vi "LVClass_CorrectionDataManager GetWavefrontCorrectorInitialPreferences.vi"(0 "CorrectionDataManager in":refnum<class "CorrectionDataManager.lvclass">, 11 "error in (no error)":errorcluster) -> (4 "CorrectionDataManager out":refnum<class "CorrectionDataManager.lvclass">, 8 "Wavefront Corrector State":T1[](array[typedef]), 15 "error out":errorcluster)   [LabVIEW 2020, in "CorrectionDataManager.lvclass"]
doc: "--------------------------------------------------------------------------------\n\n<B>corrdata_managerIn </B> : CorrDataManager object\n<B>corrdata_managerOut </B> : CorrDataManager object\n<B>min </B> : WavefrontCorrector preferences : lowest command value.\n<B>max </B> : WavefrontCorrector preferences : highest command value.\n<B>validity </B> : WavefrontCorrector preferences : status.\n<B>fixed_value </B> : WavefrontCorrector preferences : fixed positions.\n<B>ErrorIn </B> : Error\n<B>ErrorOut </B> : Error\n\n--------------------------------------------------------------------------------"
uses:
  CorrectionDataManager.lvclass
  Wavefront Corrector states - ONE.ctl
  CorrectionDataManager.lvclass/CorrectionDataManager.ctl
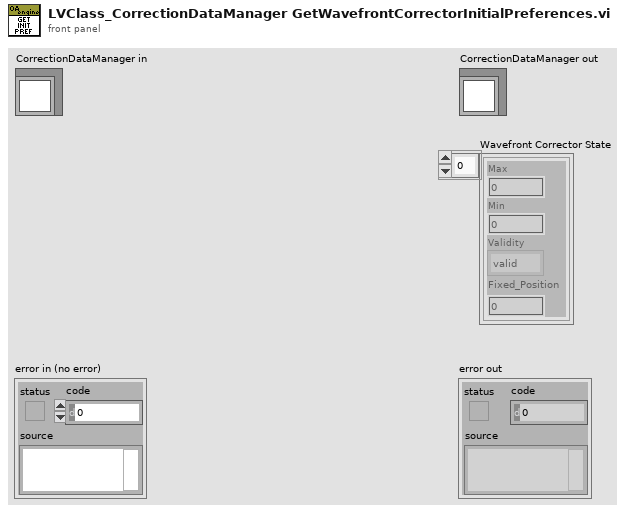
[diagram p1: front panel]
types:
  T1 = typedef "Wavefront Corrector states - ONE.ctl" = cluster{"Max":sgl, "Min":sgl, "Validity":enum16{"valid", "fixed", "invalid"}, "Fixed_Position":sgl}
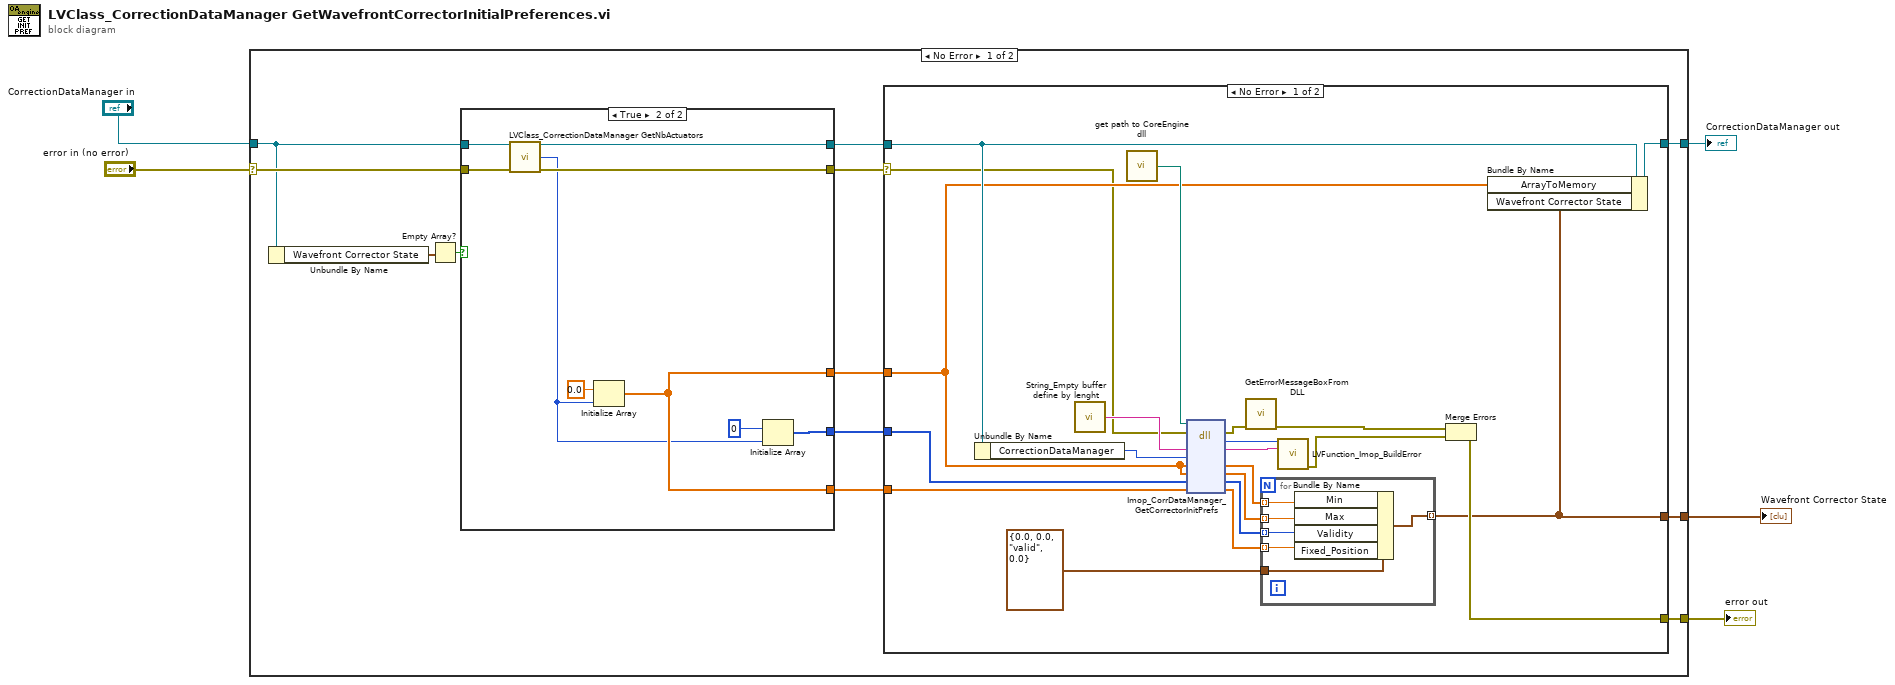
[diagram p0: block diagram]
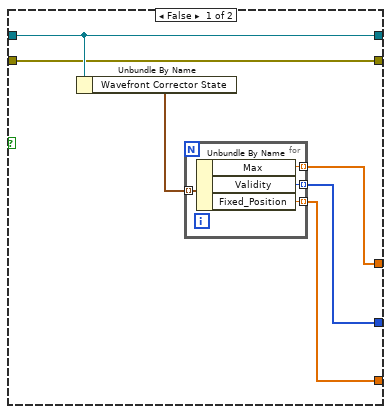
[diagram p3: hidden frame]
diagram:
  n1 = case shown="No Error" "error in (no error)" {
    selector: "error in (no error)" -> [w14 w67]
    tunnel: [w17 w67] -> w4
    tunnel: [w9 w66] -> w5
    tunnel: "CorrectionDataManager in" -> [w13 w66]
    tunnel: [w8 _] -> w1
    frame No Error {
      n2 = Unbundle By Name(w13) -> ("Wavefront Corrector State"=w16:T1[])
      n3 = Empty Array?(array=w16) -> (empty?=w15:bool)
      n4 = case shown="True" w15 {
        tunnel: w13 -> [w52 w63]
        tunnel: [w52 w57] -> w10
        tunnel: [w50 w59] -> w7
        tunnel: [w48 w59] -> w12
        tunnel: w14 -> [w51 w62]
        tunnel: [w51 w61] -> w6
        tunnel: [w49 w60] -> w11
        frame False {
          n5 = Unbundle By Name(w52) -> ("Wavefront Corrector State"=w47:T1[])
          n6 = for {
            tunnel: w47 -> [w56] mode=indexing
            tunnel: [w55] -> w50 mode=indexing
            tunnel: [w54] -> w49 mode=indexing
            tunnel: [w53] -> w48 mode=indexing
            n7 = Unbundle By Name(w56) -> ("Max"=w55:sgl, "Validity"=w54:enum16{"valid", "fixed", "invalid"}, "Fixed_Position"=w53:sgl)
          }
        }
        frame True {
          n8 = call "LVClass_CorrectionDataManager GetNbActuators.vi"("CorrectionDataManager in"=w63, "error in (no error)"=w62) -> ("CorrectionDataManager out"=w57:refnum<class "CorrectionDataManager.lvclass">, "Nb actuators"=w58:i32, "error out"=w61:errorcluster)  [unwired: 11 in]
          n9 = Initialize Array(sgl 0.0, w58) -> (w59:sgl[])
          n10 = Initialize Array(0, w58) -> (w60:i32[])
        }
      }
      n11 = case shown="No Error" w6 {
        selector: w6 -> [w18 w46]
        tunnel: [w31 w46] -> w17
        tunnel: w12 -> [w25 _]
        tunnel: w11 -> [w24 _]
        tunnel: w10 -> [w23 w45]
        tunnel: [w22 w45] -> w9
        tunnel: [w21 _] -> w8
        tunnel: w7 -> [w19 _]
        frame No Error {
          n12 = Unbundle By Name(w23) -> ("CorrectionDataManager"=w30:i32)
          n13 = call "String_Empty buffer define by lenght.vi"() -> ("Empty buffer"=w36:string)  [unwired: 1 in]
          n14 = call "get path to CoreEngine dll.vi"() -> ("path to c_interface_vc100.dll"=w35:path)  [unwired: 12 in, 3 out]
          n15 = dll-call lib="D:/soft/HASO_v3/SVN_trunk/ImOpCoreEngine4_LV2011/DLLs/c_interface_vc100.dll" fn="Imop_CorrDataManager_GetCorrectorInitPrefs"(path in=w35, error in=w18, "message"=w36, "WavefrontCorrection"=w30, "min"=w19, "max"=w19, "validity"=w24, "fixed_value"=w25) -> (error out=w34:errorcluster, "return type"=w38:i32, "message"=w37:string, "min"=w29:sgl[], "max"=w28:sgl[], "validity"=w27:i32[], "fixed_value"=w26:sgl[])  [unwired: 2 in, 1 out]
          n16 = call "GetErrorMessageBoxFromDLL.vi"("error IN"=w34) -> ("error OUT"=w33:errorcluster)  [unwired: 10 in]
          n17 = for {
            tunnel: w29 -> [w39] mode=indexing
            tunnel: w28 -> [w40] mode=indexing
            tunnel: w27 -> [w44] mode=indexing
            tunnel: w26 -> [w43] mode=indexing
            tunnel: [w42] -> w21 mode=indexing
            tunnel: T1 {"Max"=0.0, "Min"=0.0, "Validity"=enum."valid", "Fixed_Position"=0.0} ("Actuator state") -> [w41]
            n18 = Bundle By Name(cluster=w41, "Min"=w39, "Max"=w40, "Validity"=w44, "Fixed_Position"=w43) -> (w42:T1)
          }
          n19 = call "LVFunction_Imop_BuildError.vi"("code"=w38, "String to Prepend to source (\"\")"=w37) -> ("error out"=w32:errorcluster)  [unwired: 13 in]
          n20 = Merge Errors(w33, w32) -> (w31:errorcluster)
          n21 = Bundle By Name(cluster=w23, "ArrayToMemory"=w19, "Wavefront Corrector State"=w21) -> (w22:refnum<class "CorrectionDataManager.lvclass">)
        }
        frame Error {
        }
      }
    }
    frame Error {
    }
  }
  "error out" <- w4
  "CorrectionDataManager out" <- w5
  "Wavefront Corrector State" <- w1
